vi "dotNET Parse UI Details.vi"(8 "error in":errorcluster) -> (0 "error out":errorcluster, 3 "Measurement UI Details":T1)   [LabVIEW 2020, in "Measurement Client Wrapper.lvclass"]
uses:
  Measurement Client Wrapper.lvclass
  Typedefs/Measurement UI Details.ctl
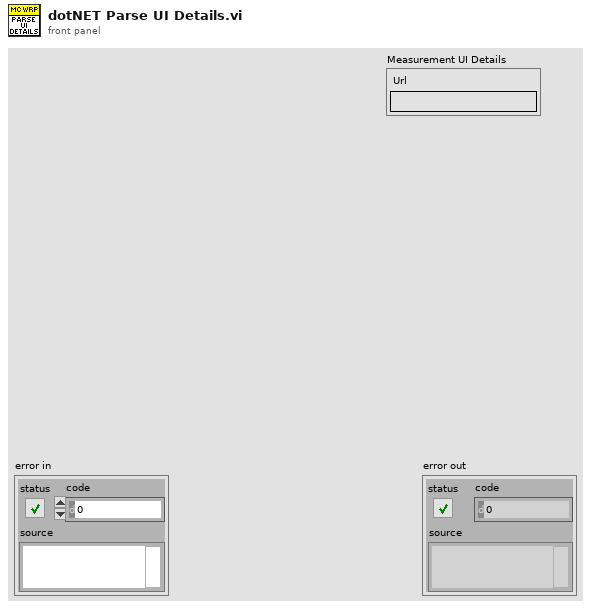
[diagram p1: front panel]
types:
  T1 = typedef "Measurement Client Wrapper.lvclass/Measurement UI Details.ctl" = cluster{"Url":string}
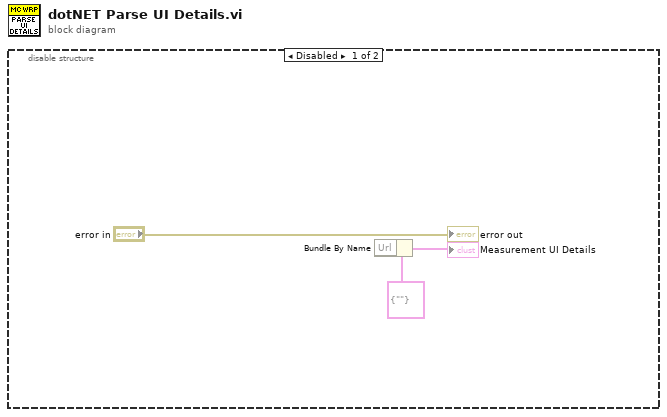
[diagram p0: block diagram]
diagram:
  n1 = disable-structure shown="Disabled" {
    frame Disabled {
      n2 = Bundle By Name(cluster=T1 {"Url"=""} ("Measurement UI Details")) -> (→"Measurement UI Details":T1)  [unwired: 1 in]
      "error out" <- "error in"
    }
    frame Enabled {
    }
  }
